vi "Switch all lasers.vi"(8 "error in":errorcluster, 9 "Live channel":enum8{"Red", "Green", "Blue", "UV", ""}(ring)=enum."", 10 "Lasers connected?":bool=TRUE, 11 "Laser cluster":T1) -> (0 "error out":errorcluster)   [LabVIEW 2017]
panel:
  in  "Switching delay (ms)":u32=200
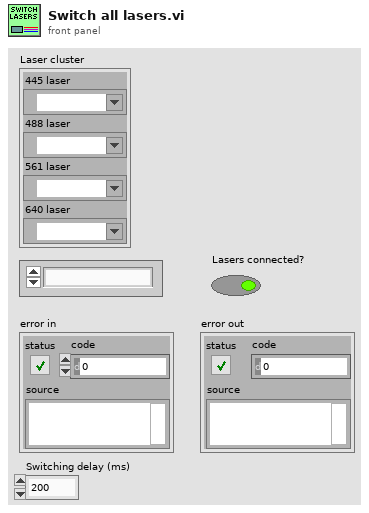
[diagram p1: front panel]
types:
  T1 = cluster{"445 laser":refnum<visa-resource-name>, "488 laser":refnum<visa-resource-name>, "561 laser":refnum<visa-resource-name>, "640 laser":refnum<visa-resource-name>}
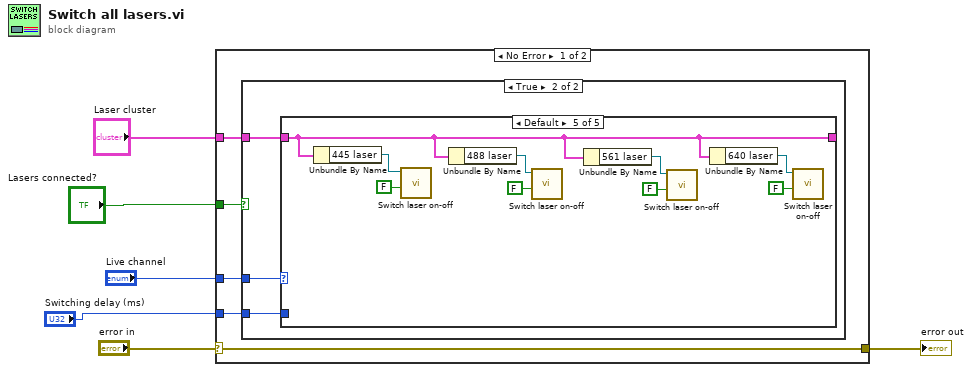
[diagram p0: block diagram]
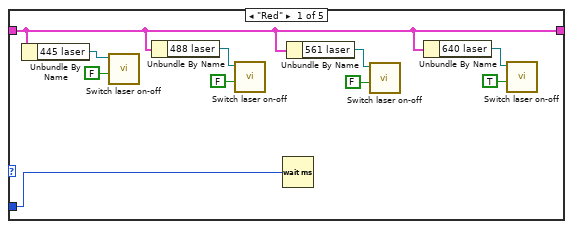
[diagram p3: hidden frame]
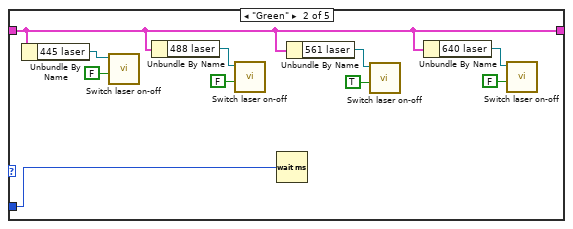
[diagram p4: hidden frame]
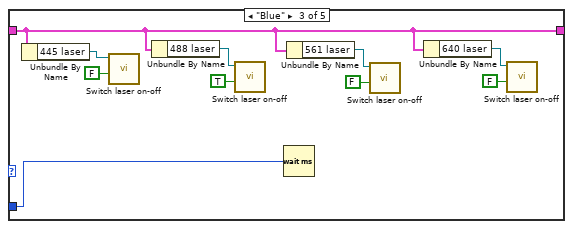
[diagram p5: hidden frame]
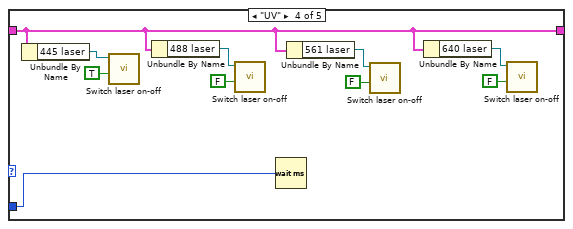
[diagram p6: hidden frame]
diagram:
  n1 = case shown="No Error" "error in" {
    selector: "error in" -> [w8 w64]
    tunnel: "Live channel" -> [w11 _]
    tunnel: "Laser cluster" -> [w10 _]
    tunnel: "Lasers connected?" -> [w9 _]
    tunnel: [w8 w64] -> w2
    tunnel: "Switching delay (ms)" -> [w7 _]
    frame No Error {
      n2 = case shown="True" w9 {
        tunnel: w11 -> [_ w14]
        tunnel: w10 -> [_ w13]
        tunnel: w7 -> [_ w12]
        frame False {
        }
        frame True {
          n3 = case shown="Default" w14 {
            tunnel: w13 -> [w20 w30 w40 w50 w59]
            tunnel: [w20 w30 w40 w50 w59] -> _
            tunnel: w12 -> [w15 w25 w35 w45 _]
            frame "Red" {
              n4 = Unbundle By Name(w20) -> ("445 laser"=w24:refnum<visa-resource-name>)
              n5 = call "Switch laser on-off.vi"("Laser On/Off"=FALSE, "VISA resource name"=w24) -> ()  [unwired: 9 in, 1 out]
              n6 = Unbundle By Name(w20) -> ("488 laser"=w23:refnum<visa-resource-name>)
              n7 = call "Switch laser on-off.vi"("Laser On/Off"=FALSE, "VISA resource name"=w23) -> ()  [unwired: 9 in, 1 out]
              n8 = Wait (ms)(milliseconds to wait=w15) -> ()  [unwired: 1 out]
              n9 = Unbundle By Name(w20) -> ("561 laser"=w22:refnum<visa-resource-name>)
              n10 = call "Switch laser on-off.vi"("Laser On/Off"=FALSE, "VISA resource name"=w22) -> ()  [unwired: 9 in, 1 out]
              n11 = Unbundle By Name(w20) -> ("640 laser"=w21:refnum<visa-resource-name>)
              n12 = call "Switch laser on-off.vi"("Laser On/Off"=TRUE, "VISA resource name"=w21) -> ()  [unwired: 9 in, 1 out]
            }
            frame "Green" {
              n13 = Unbundle By Name(w30) -> ("445 laser"=w34:refnum<visa-resource-name>)
              n14 = call "Switch laser on-off.vi"("Laser On/Off"=FALSE, "VISA resource name"=w34) -> ()  [unwired: 9 in, 1 out]
              n15 = Unbundle By Name(w30) -> ("488 laser"=w33:refnum<visa-resource-name>)
              n16 = call "Switch laser on-off.vi"("Laser On/Off"=FALSE, "VISA resource name"=w33) -> ()  [unwired: 9 in, 1 out]
              n17 = Wait (ms)(milliseconds to wait=w25) -> ()  [unwired: 1 out]
              n18 = Unbundle By Name(w30) -> ("561 laser"=w32:refnum<visa-resource-name>)
              n19 = call "Switch laser on-off.vi"("Laser On/Off"=TRUE, "VISA resource name"=w32) -> ()  [unwired: 9 in, 1 out]
              n20 = Unbundle By Name(w30) -> ("640 laser"=w31:refnum<visa-resource-name>)
              n21 = call "Switch laser on-off.vi"("Laser On/Off"=FALSE, "VISA resource name"=w31) -> ()  [unwired: 9 in, 1 out]
            }
            frame "Blue" {
              n22 = Unbundle By Name(w40) -> ("445 laser"=w44:refnum<visa-resource-name>)
              n23 = call "Switch laser on-off.vi"("Laser On/Off"=FALSE, "VISA resource name"=w44) -> ()  [unwired: 9 in, 1 out]
              n24 = Unbundle By Name(w40) -> ("488 laser"=w43:refnum<visa-resource-name>)
              n25 = call "Switch laser on-off.vi"("Laser On/Off"=TRUE, "VISA resource name"=w43) -> ()  [unwired: 9 in, 1 out]
              n26 = Wait (ms)(milliseconds to wait=w35) -> ()  [unwired: 1 out]
              n27 = Unbundle By Name(w40) -> ("561 laser"=w42:refnum<visa-resource-name>)
              n28 = call "Switch laser on-off.vi"("Laser On/Off"=FALSE, "VISA resource name"=w42) -> ()  [unwired: 9 in, 1 out]
              n29 = Unbundle By Name(w40) -> ("640 laser"=w41:refnum<visa-resource-name>)
              n30 = call "Switch laser on-off.vi"("Laser On/Off"=FALSE, "VISA resource name"=w41) -> ()  [unwired: 9 in, 1 out]
            }
            frame "UV" {
              n31 = Unbundle By Name(w50) -> ("445 laser"=w54:refnum<visa-resource-name>)
              n32 = call "Switch laser on-off.vi"("Laser On/Off"=TRUE, "VISA resource name"=w54) -> ()  [unwired: 9 in, 1 out]
              n33 = Unbundle By Name(w50) -> ("488 laser"=w53:refnum<visa-resource-name>)
              n34 = call "Switch laser on-off.vi"("Laser On/Off"=FALSE, "VISA resource name"=w53) -> ()  [unwired: 9 in, 1 out]
              n35 = Wait (ms)(milliseconds to wait=w45) -> ()  [unwired: 1 out]
              n36 = Unbundle By Name(w50) -> ("561 laser"=w52:refnum<visa-resource-name>)
              n37 = call "Switch laser on-off.vi"("Laser On/Off"=FALSE, "VISA resource name"=w52) -> ()  [unwired: 9 in, 1 out]
              n38 = Unbundle By Name(w50) -> ("640 laser"=w51:refnum<visa-resource-name>)
              n39 = call "Switch laser on-off.vi"("Laser On/Off"=FALSE, "VISA resource name"=w51) -> ()  [unwired: 9 in, 1 out]
            }
            frame Default {
              n40 = Unbundle By Name(w59) -> ("445 laser"=w63:refnum<visa-resource-name>)
              n41 = call "Switch laser on-off.vi"("Laser On/Off"=FALSE, "VISA resource name"=w63) -> ()  [unwired: 9 in, 1 out]
              n42 = Unbundle By Name(w59) -> ("488 laser"=w62:refnum<visa-resource-name>)
              n43 = call "Switch laser on-off.vi"("Laser On/Off"=FALSE, "VISA resource name"=w62) -> ()  [unwired: 9 in, 1 out]
              n44 = Unbundle By Name(w59) -> ("561 laser"=w61:refnum<visa-resource-name>)
              n45 = call "Switch laser on-off.vi"("Laser On/Off"=FALSE, "VISA resource name"=w61) -> ()  [unwired: 9 in, 1 out]
              n46 = Unbundle By Name(w59) -> ("640 laser"=w60:refnum<visa-resource-name>)
              n47 = call "Switch laser on-off.vi"("Laser On/Off"=FALSE, "VISA resource name"=w60) -> ()  [unwired: 9 in, 1 out]
            }
          }
        }
      }
    }
    frame Error {
    }
  }
  "error out" <- w2
